vi "KBackground Gradient Test.vi"() -> ()   [LabVIEW 2015]
uses:
  KBackground Gradient/KBackground Gradient.xctl
panel:
  in  "KBackground Gradient":dbl(xcontrol)
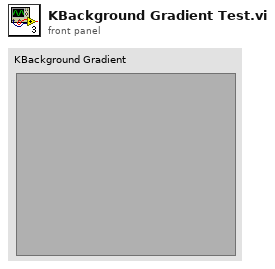
[diagram p1: front panel]
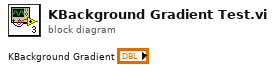
[diagram p0: block diagram]
diagram:
